vi "From Variant.vi"(8 "error in (no error)":errorcluster, 11 "Variant":variant) -> (0 "error out":errorcluster, 3 "Boolean out":refnum<class "Path.lvclass">)   [LabVIEW 2019, in "Path.lvclass"]
uses:
  <vilib>/gpm_packages/@cs/data-type-serializer/source/Path/Path.lvclass
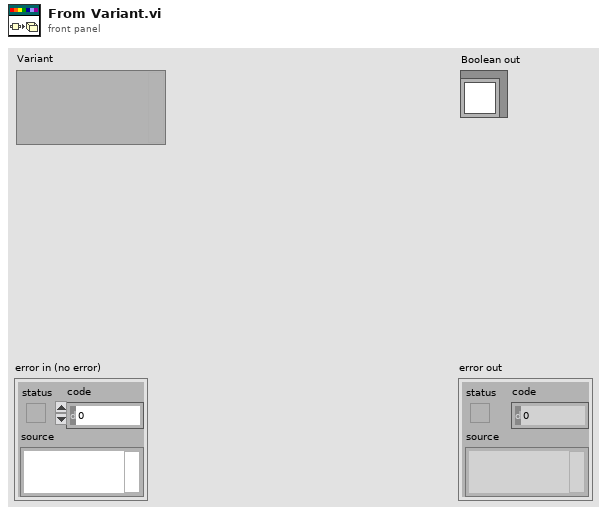
[diagram p1: front panel]
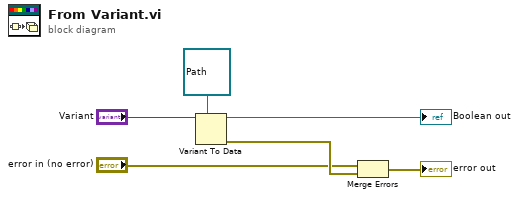
[diagram p0: block diagram]
diagram:
  n1 = Variant To Data(type=refnum<class "Path.lvclass"> refnum ("Boolean in"), Variant="Variant") -> (data=→"Boolean out":refnum<class "Path.lvclass">, error out=w5:errorcluster)  [unwired: 1 in]
  n2 = Merge Errors("error in (no error)", w5) -> (→"error out":errorcluster)
